vi "ADAM_scan_diagnostic.vi"() -> ()   [LabVIEW 2010]
uses:
  ADAM Client/Sub VIs/ADAM Controls/Ch_description_ADAM.ctl
  ADAM Client/Sub VIs/ADAM Controls/Module_type_ADAM.ctl
  ADAM Client/Sub VIs/ADAM Controls/Function_ADAM.ctl
  ADAM Client/Sub VIs/ADAM Controls/Channel_State.ctl
  ADAM Client/Sub VIs/ADAM Controls/Calib_type_ADAM.ctl
  ADAM Client/Sub VIs/ADAM Controls/Address.ctl
  Sub VI's/Channel_Description_Global.vi
  ADAM_Global.vi
panel:
  in  "Save Changes":bool
  out "Index":i32
  in  "Simulate":bool
  in  "stop":bool
  in  "Value to Output":dbl format="%.2f"
  out "Calibrated units":dbl format="%.2f"
  out "Scan comment":string
  in  "Execute channel":bool
  in  "Select channel":bool
  in  "Ch Description":T1 {"Duty" format="%.0b"; "D" format="%#_5g"; "C" format="%#_5g"; "B" format="%#_5g"; "A" format="%#_5g"}
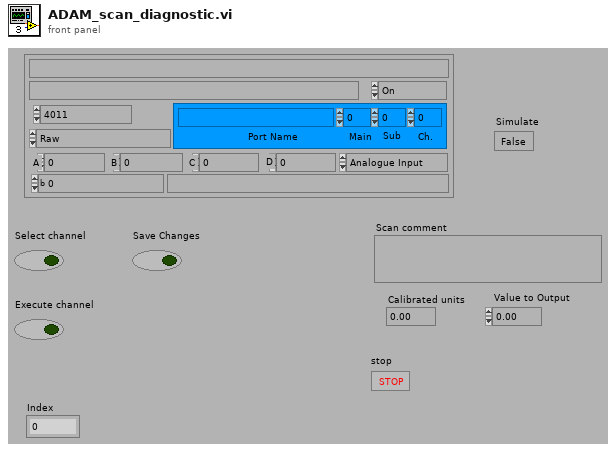
[diagram p1: front panel]
types:
  T1 = typedef "Ch_description_ADAM.ctl" = cluster{"Ch Name":string, "Type":T2, "Function":T3, "Ch State":T4, "Calibration type":T5, "A":dbl, "B":dbl, "C":dbl, "D":dbl, "Comments":string, "Address":T6, "String":string, "Duty":u16}
  T2 = typedef "Module_type_ADAM.ctl" = enum16{"4011", "4012", "4013", "4014", "4016", "4017", "4018", "4021", "4050", "4052", "4053", "4060", "4080", "5000", "5017", "5018", "5024", "5051", "5056", "5060", "6060", "Tracker", "WEST", "GILL", "JEM", "VICI", "Vaisala", "DRUCK", "Run VI Named:", "IR2100", "PPT", "Comparator", "VIRTUAL", "Hold Value", "Read A", "Read Ch", "Coded", "Client Info", "Web Client", "X10", "Test"}
  T3 = typedef "Function_ADAM.ctl" = enum16{"Analogue Input", "Digital Input", "Event counter", "Event rate", "Analogue Output", "Digital Output", "Relay Output"}
  T4 = typedef "Channel_State.ctl" = enum16{"On", "Off", "Always On", "Always Off"}
  T5 = typedef "Calib_type_ADAM.ctl" = enum16{"Raw", "Bx + A", "Cx^2 + Bx + A", "Dx^3 + Cx^2 + Bx + A", "In Band", "Hi-Tec Q", "Hi-Tec M_dot", "Text"}
  T6 = typedef "Address.ctl" = cluster{"Main":i32, "Ch.":i32, "Sub":i32, "Port Name":string}
  T7 = enum16{"Load ADAM setup from excel file", "Save ADAM setup to excel file"}
  T8 = enum16{"Zero or one", "One", "Zero or more", "One or more"}
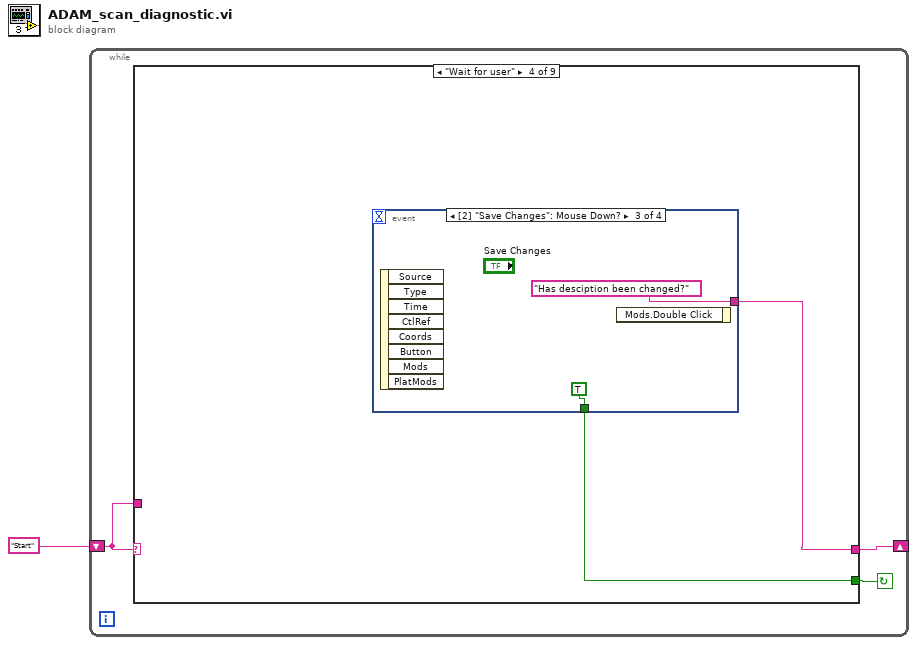
[diagram p0: block diagram]
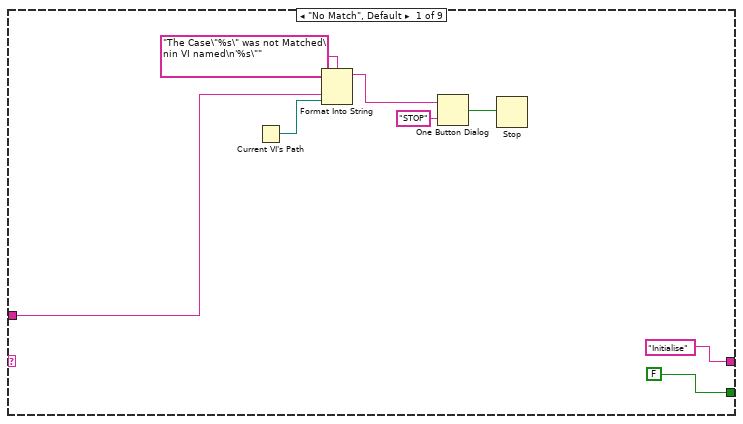
[diagram p2: hidden frame]
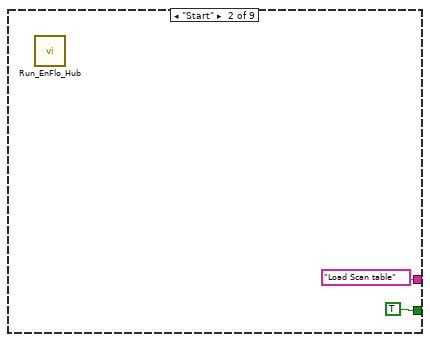
[diagram p3: hidden frame]
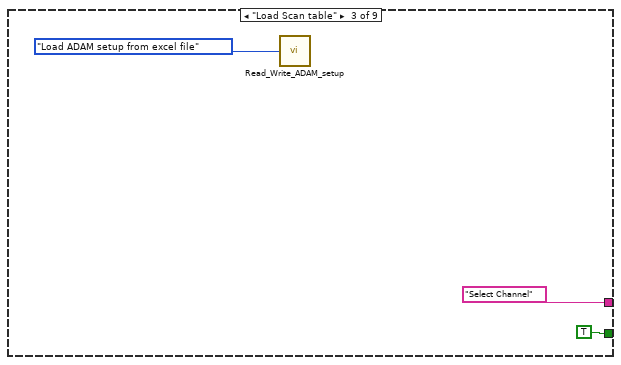
[diagram p4: hidden frame]
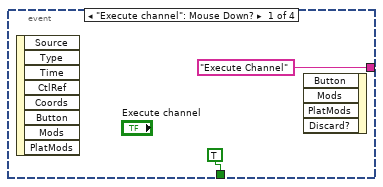
[diagram p5: hidden frame]
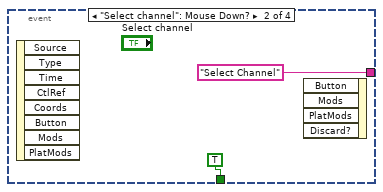
[diagram p6: hidden frame]
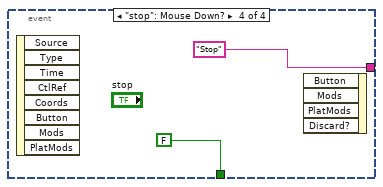
[diagram p7: hidden frame]
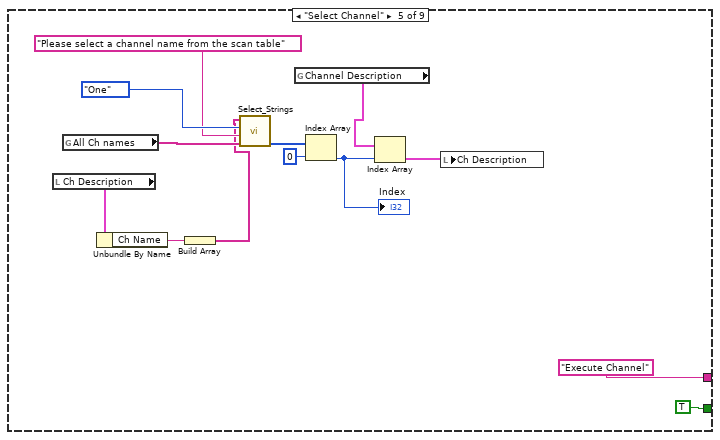
[diagram p8: hidden frame]
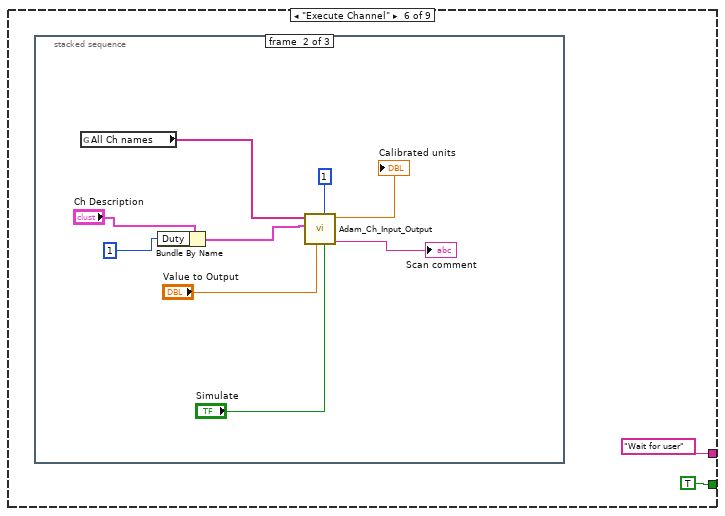
[diagram p9: hidden frame]
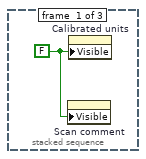
[diagram p10: hidden frame]
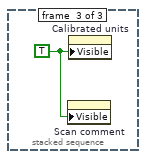
[diagram p11: hidden frame]
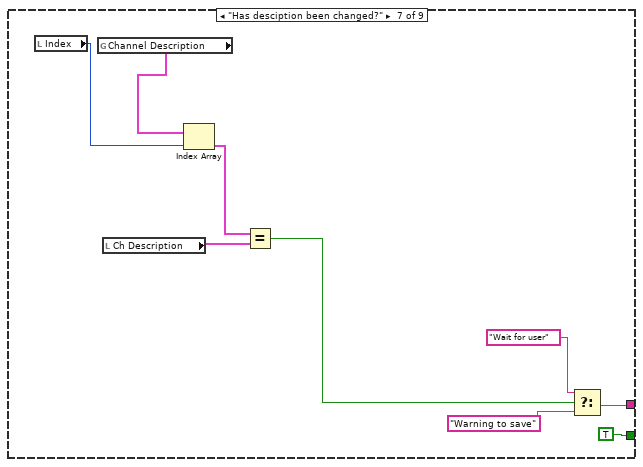
[diagram p12: hidden frame]
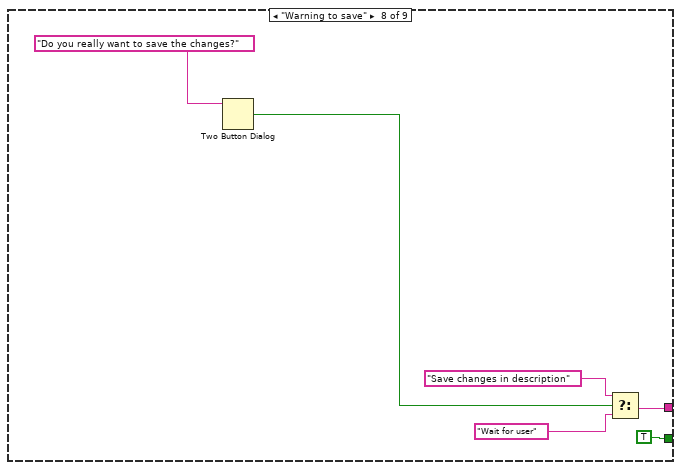
[diagram p13: hidden frame]
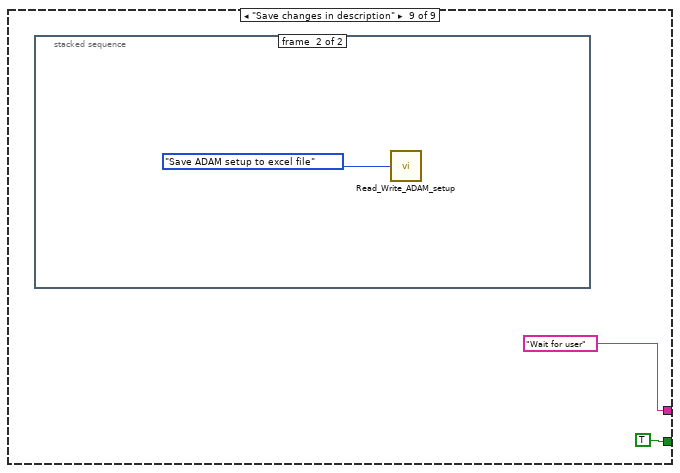
[diagram p14: hidden frame]
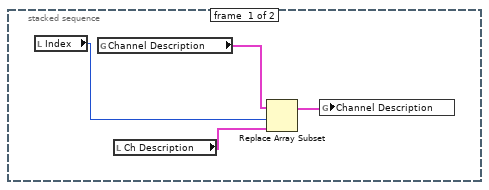
[diagram p15: hidden frame]
diagram:
  n1 = while {
    shift-left: "Start" -> [w2]
    shift-right: [w3] -> _
    stop <- w4 continue-if-true
    n2 = case shown="\"Wait for user\"" w2 {
      tunnel: [FALSE TRUE TRUE w18 TRUE TRUE TRUE TRUE TRUE] -> w4
      tunnel: ["Initialise" "Load Scan table" "Select Channel" w19 "Execute Channel" "Wait for user" w55 w67 "Wait for user"] -> w3
      tunnel: w2 -> [w7 _ _ _ _ _ _ _ _]
      frame "No Match", Default {
        n3 = Current VI's Path() -> (path=w6:path)
        n4 = Format Into String(format string="The Case\"%s\" was not Matched\nin VI named\n'%s\"" ("Format String"), w7, w6) -> (resulting string=w10:string)  [unwired: 2 in, 1 out]
        n5 = One Button Dialog(message=w10, button name ("OK")="STOP") -> (true=w8:bool)
        n6 = Stop(stop? (T)=w8) -> ()
      }
      frame "Start" {
        n7 = call "Run_EnFlo_Hub.vi"() -> ()  [unwired: 8 in]
      }
      frame "Load Scan table" {
        n8 = call "Read_Write_ADAM_setup.vi"("Mode"=T7."Load ADAM setup from excel file") -> ()  [unwired: 4 in]
      }
      frame "Wait for user" {
        n9 = event shown="[2] \"Save Changes\": Mouse Down?" {
          selector: _ -> [_ _ _ _]
          dyn-events: _ -> [_ _ _ _]
          timeout: _ -> [_ _ _ _]
          tunnel: ["Execute Channel" "Select Channel" "Has desciption been changed?" "Stop"] -> w19
          tunnel: [TRUE TRUE TRUE FALSE] -> w18
          event "Execute channel": Mouse Down? {
            n10 = event-data() -> ()  [unwired: 1 in, 8 out]
            n11 = event-data() -> ()  [unwired: 5 in, 1 out]
          }
          event "Select channel": Mouse Down? {
            n12 = event-data() -> ()  [unwired: 1 in, 8 out]
            n13 = event-data() -> ()  [unwired: 5 in, 1 out]
          }
          event "Save Changes": Mouse Down? {
            n14 = event-data() -> ()  [unwired: 1 in, 8 out]
            n15 = event-data() -> ()  [unwired: 2 in, 1 out]
          }
          event "stop": Mouse Down? {
            n16 = event-data() -> ()  [unwired: 1 in, 8 out]
            n17 = event-data() -> ()  [unwired: 5 in, 1 out]
          }
        }
      }
      frame "Select Channel" {
        n18 = local read "Ch Description"() -> (w30:T1)
        n19 = global read "ADAM_Global.vi" "All Ch names"() -> (w38:string[])
        n20 = Unbundle By Name(w30) -> ("Ch Name"=w29:string)
        n21 = Build Array(w29) -> (w28:string[])
        n22 = call "Select_Strings.vi"("Available Ch names"=w38, "Message"="Please select a channel name from the scan table", "Selector mode"=T8."One", "Desired Ch names (in)"=w28) -> ("Ch Indicies Choosen"=w34:i32[])  [unwired: 2 in, 2 out]
        n23 = global read "Channel_Description_Global.vi" "Channel Description"() -> (w32:T1[])
        n24 = Index Array(array=w34, index=0) -> (element=w33:i32)
        "Index" <- w33
        n25 = Index Array(array=w32, index=w33) -> (element=w31:T1)
        n26 = local write "Ch Description"(w31) -> ()
      }
      frame "Execute Channel" {
        n27 = stacked-sequence {
          frame #0 {
            w43 = FALSE ("Visible")
            n28 = property on="Scan comment" class="Str"("Visible"=w43) -> ()  [unwired: 2 in, 2 out]
            n29 = property on="Calibrated units" class="DigNum (strict)"("Visible"=w43) -> ()  [unwired: 2 in, 2 out]
          }
          frame #1 {
            n30 = global read "ADAM_Global.vi" "All Ch names"() -> (w46:string[])
            n31 = Bundle By Name(cluster="Ch Description", "Duty"=u16 1 ("Duty No")) -> (w47:T1)
            n32 = call "Adam_Ch_Input_Output.vi"("Simulate"="Simulate", "Duty No"=u16 1, "Value to Output"="Value to Output", "Ch Discription"=w47, "Ch names"=w46) -> ("Scan comment"=→"Scan comment":string, "Calibrated units"=→"Calibrated units":dbl)  [unwired: 5 in]
          }
          frame #2 {
            w53 = TRUE ("Visible")
            n33 = property on="Scan comment" class="Str"("Visible"=w53) -> ()  [unwired: 2 in, 2 out]
            n34 = property on="Calibrated units" class="DigNum (strict)"("Visible"=w53) -> ()  [unwired: 2 in, 2 out]
          }
        }
      }
      frame "Has desciption been changed?" {
        n35 = local read "Index"() -> (w61:i32)
        n36 = global read "Channel_Description_Global.vi" "Channel Description"() -> (w60:T1[])
        n37 = local read "Ch Description"() -> (w58:T1)
        n38 = Index Array(array=w60, index=w61) -> (element=w59:T1)
        n39 = Equal?(x=w59, y=w58) -> (x = y?=w57:bool)
        n40 = Select(t="Wait for user", s=w57, f="Warning to save") -> (s? t:f=w55:string)
      }
      frame "Warning to save" {
        n41 = Two Button Dialog(message="Do you really want to save the changes?") -> (T button?=w65:bool)  [unwired: 2 in]
        n42 = Select(t="Save changes in description" ("f"), s=w65, f="Wait for user") -> (s? t:f=w67:string)
      }
      frame "Save changes in description" {
        n43 = stacked-sequence {
          frame #0 {
            n44 = local read "Index"() -> (w73:i32)
            n45 = global read "Channel_Description_Global.vi" "Channel Description"() -> (w74:T1[])
            n46 = local read "Ch Description"() -> (w72:T1)
            n47 = Replace Array Subset(array=w74, new element=w72, index=w73) -> (w71:T1[])
            n48 = global write "Channel_Description_Global.vi" "Channel Description"(w71) -> ()
          }
          frame #1 {
            n49 = call "Read_Write_ADAM_setup.vi"("Mode"=T7."Save ADAM setup to excel file") -> ()  [unwired: 4 in]
          }
        }
      }
    }
  }
